vi "UE9 Synchronized Stream Example.vi"() -> ()   [LabVIEW 2021]
panel:
  out "UD Backlog B":i32
  out "UD Backlog A":i32
  in  "AIN Range":u16(ring) items=["LJ_rgBIP5V", "LJ_rgUNI5V", "LJ_rgUNI2P5V", "LJ_rgUNI1P25V", "LJ_rgUNIP625V"]
  out "Data B":dbl[][](array[numeric]) format="%.3f"
  out "Comm Backlog B":i32
  out "# Scans Read B":i32
  in  "Sync Wire Installed":bool=TRUE
  in  "Address B":string="3"
  out "Actual Scan Rate (Hz)":dbl=1000.0 format="%.3f"
  out "ms Per Loop":u32
  out "Comm Backlog A":i32
  out "# Scans Read A":i32
  out "# of iterations":i32
  out "Data A":dbl[][](array[numeric]) format="%.3f"
  in  "Scan Rate (Hz)":dbl=1000.0 format="%.3f"
  in  "Scan List":u8[](array[numeric])=[0, 1, 2, 3]
  in  "stop":bool
  in  "ConnectionType":u16(ring) items=["LJ_ctUSB", "LJ_ctETHERNET"]
  in  "Address A":string="2"
  out "Error Message":string
  in  "Resolution":i32=12
  # "Demonstrates synchronized streaming with 2 UE9s.  Connect FIO0 on unit A to FIO0 on unit B.  If the units are isolated from each other, generally\nmeaning no USB cables, you should also connect GND to GND.  Note that\tthe external clock input or output uses FIO0 in this example since no\nother timers or counters are enabled.  The external clock uses\tCounter1, so if any other timers or counters are enabled, the external\nstream clock will be on the next available FIO line, as Counter1 is always last.  If using other timer/counters, it is recommended that\nthey be configured before the stream."
  # "Specify an IP address\nfor Ethernet, or Local\nID for USB."
  # "Select if a FIO0 is connected between\nunit A and unit B.  Otherwise, the two\nunits will stream at the same time, but\nare not synchronized.  That means the\ntimes they both start streaming will\ndiffer by the time to start a stream (a\nfew milliseconds), and over time there\nwill likely be drift as the units do not\nhave the same clock."
  # "This example uses the same\nscan list for both units."
  # "(for all channels)"
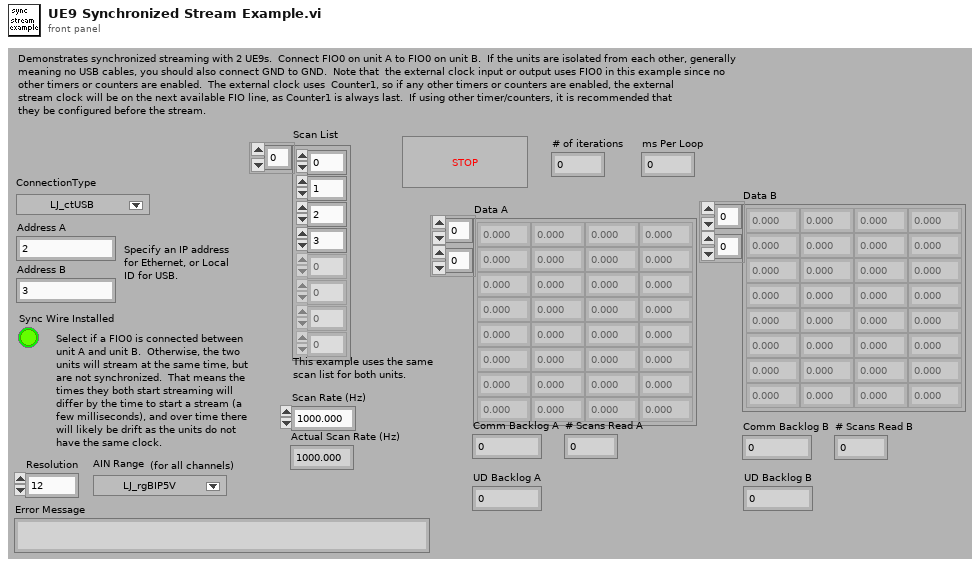
[diagram p1: front panel]
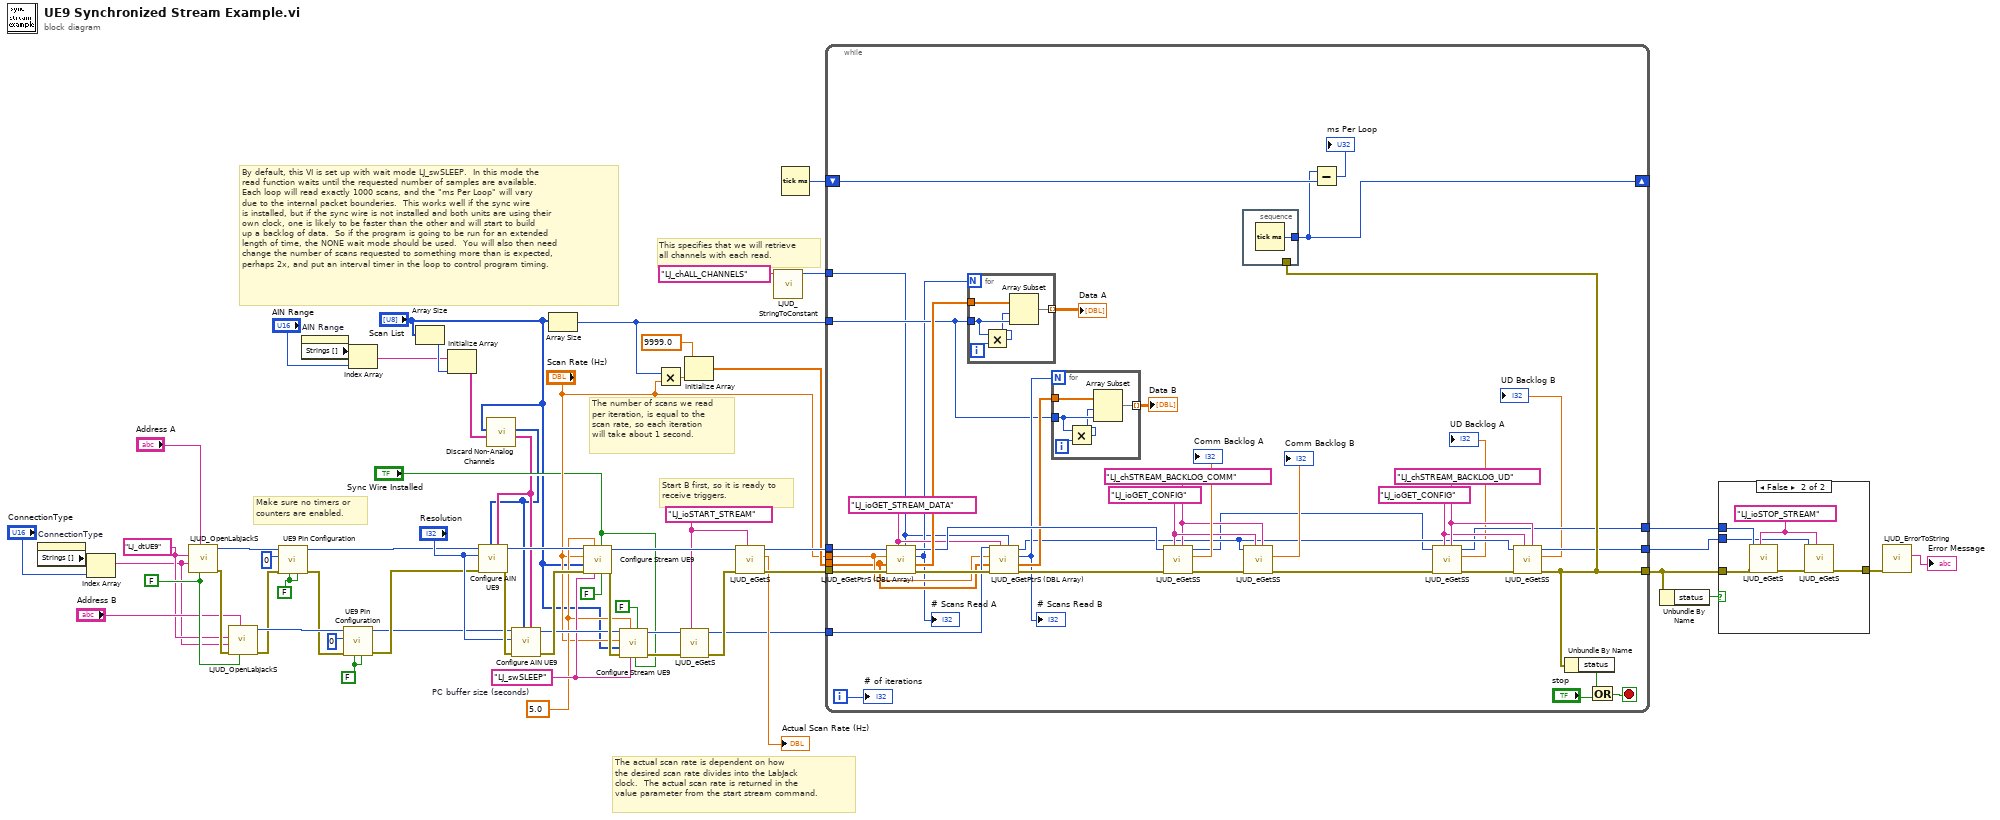
[diagram p0: block diagram]
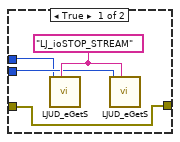
[diagram p2: hidden frame]
diagram:
  w34 = "LJ_swSLEEP" ("Wait Mode")
  w15 = "LJ_dtUE9" ("DeviceType")
  w23 = FALSE ("Enable Counter0")
  w26 = FALSE ("Enable Counter0")
  w37 = FALSE ("FirstFound")
  w33 = 5.0  # PC buffer size (seconds)
  w47 = "LJ_ioSTART_STREAM" ("IOType")
  # "This specifies that we will retrieve\nall channels with each read."
  # "Make sure no timers or\ncounters are enabled."
  # "Start B first, so it is ready to\nreceive triggers."
  # "The actual scan rate is dependent on how\nthe desired scan rate divides into the LabJack\nclock.  The actual scan rate is returned in the\nvalue parameter from the start stream command."
  # "By default, this VI is set up with wait mode LJ_swSLEEP.  In this mode the\nread function waits until the requested number of samples are available.\nEach loop will read exactly 1000 scans, and the \"ms Per Loop\" will vary\ndue to the internal packet bounderies.  This works well if the sync wire\nis installed, but if the sync wire is not installed and both units are using their\nown clock, one is likely to be faster than the other and will start to build\nup a backlog of data.  So if the program is going to be run for an extended\nlength of time, the NONE wait mode should be used.  You will also then need\nchange the number of scans requested to something more than is expected,\nperhaps 2x, and put an interval timer in the loop to control program timing."
  # "The number of scans we read\nper iteration, is equal to the\nscan rate, so each iteration\nwill take about 1 second."
  n1 = property on="ConnectionType" class="Ring (strict)"() -> ("Strings []"=w14:string[])  [unwired: 2 in, 2 out]
  n2 = Index Array(array=w14, index="ConnectionType") -> (element=w12:string)
  n3 = call "LJUD_OpenLabJackS.vi"("FirstFound"=w37, "Address"="Address A", "ConnectionType"=w12, "DeviceType"=w15) -> ("error out"=w46:errorcluster, "Handle"=w22:i32)  [unwired: 5 in, 1 out]
  n4 = call "LJUD_OpenLabJackS.vi"("FirstFound"=w37, "Address"="Address B", "error in"=w46, "ConnectionType"=w12, "DeviceType"=w15) -> ("error out"=w20:errorcluster, "Handle"=w21:i32)  [unwired: 4 in, 1 out]
  n5 = call "UE9 Pin Configuration.vi"("Enable Counter1"=w26, "Enable Counter0"=w26, "error in"=w20, "Number of Timers Enabled"=u8 0 ("# Timers Enabled"), "Handle In"=w22) -> ("error out"=w19:errorcluster, "Handle Out"=w17:i32)  [unwired: 5 in]
  n6 = property on="AIN Range" class="Ring (strict)"() -> ("Strings []"=w11:string[])  [unwired: 2 in, 2 out]
  n7 = call "UE9 Pin Configuration.vi"("Enable Counter1"=w23, "Enable Counter0"=w23, "error in"=w19, "Number of Timers Enabled"=u8 0 ("# Timers Enabled"), "Handle In"=w21) -> ("error out"=w18:errorcluster, "Handle Out"=w16:i32)  [unwired: 5 in]
  n8 = Index Array(array=w11, index="AIN Range") -> (element=w9:string)
  n9 = Array Size(array="Scan List") -> (size(s)=w48:i32)
  n10 = Initialize Array(w9, w48) -> (w4:string[])
  n11 = call "Discard Non-Analog Channels.vi"("Ranges In"=w4, "Channels In"="Scan List") -> ("Ranges Out"=w3:string[], "Channels Out"=w1:i32[])  [unwired: 6 in, 2 out]
  n12 = call "Configure AIN UE9.vi"("Ranges"=w3, "Channels"=w1, "error in"=w18, "Resolution"="Resolution", "Handle In"=w17) -> ("error out"=w45:errorcluster, "Handle Out"=w49:i32)  [unwired: 5 in]
  n13 = call "Configure AIN UE9.vi"("Ranges"=w3, "Channels"=w1, "error in"=w45, "Resolution"="Resolution", "Handle In"=w16) -> ("error out"=w44:errorcluster, "Handle Out"=w40:i32)  [unwired: 5 in]
  n14 = Array Size(array="Scan List") -> (size(s)=w54:i32)
  n15 = call "Configure Stream UE9.vi"("External Scan Trigger"=FALSE ("Scan Clock Output"), "Scan Clock Output"="Sync Wire Installed", "Wait Mode"=w34, "PC buffer size (seconds)"=w33, "error in"=w44, "Scan List"="Scan List", "Scan Rate (Hz)"="Scan Rate (Hz)", "Handle In"=w49) -> ("error out"=w42:errorcluster, "Handle Out"=w60:i32)  [unwired: 1 in, 1 out]
  n16 = call "Configure Stream UE9.vi"("External Scan Trigger"="Sync Wire Installed", "Scan Clock Output"=FALSE ("External Scan Trigger"), "Wait Mode"=w34, "PC buffer size (seconds)"=w33, "error in"=w42, "Scan List"="Scan List", "Scan Rate (Hz)"="Scan Rate (Hz)", "Handle In"=w40) -> ("error out"=w43:errorcluster, "Handle Out"=w39:i32)  [unwired: 1 in, 1 out]
  n17 = Multiply(x=w54, y="Scan Rate (Hz)") -> (x*y=w57:dbl)
  n18 = call "LJUD_eGetS.vi"("IOType"=w47, "error in"=w43, "Handle In"=w39) -> ("error out"=w41:errorcluster, "Handle Out"=w38:i32)  [unwired: 6 in, 1 out]
  n19 = Initialize Array(9999.0, w57) -> (w55:dbl[])
  n20 = call "LJUD_eGetS.vi"("IOType"=w47, "error in"=w41, "Handle In"=w60) -> ("error out"=w59:errorcluster, "Value Read"=→"Actual Scan Rate (Hz)":dbl, "Handle Out"=w58:i32)  [unwired: 6 in]
  n21 = call "LJUD_StringToConstant.vi"("String"="LJ_chALL_CHANNELS") -> ("Constant Number"=w5:i32)  [unwired: 9 in, 1 out]
  n22 = Tick Count (ms)() -> (millisecond timer value=w51:u32)
  n23 = while {
    tunnel: w5 -> [w73]
    tunnel: [w67] -> w27
    tunnel: [w64] -> w28
    tunnel: w38 -> [w82]
    shift-left: w51 -> [w94]
    shift-right: [w93] -> _
    tunnel: [w68] -> w8
    tunnel: w54 -> [w76]
    tunnel: w55 -> [w80]
    tunnel: "Scan Rate (Hz)" -> [w81]
    tunnel: w59 -> [w98]
    tunnel: w58 -> [w99]
    i -> [w95]
    stop <- w90 stop-if-true
    w71 = "LJ_ioGET_CONFIG" ("IOType")
    w72 = "LJ_chSTREAM_BACKLOG_UD" ("Channel")
    w88 = "LJ_ioGET_CONFIG" ("IOType")
    w87 = "LJ_chSTREAM_BACKLOG_COMM" ("Channel")
    w79 = "LJ_ioGET_STREAM_DATA" ("IOType")
    n24 = call "LJUD_eGetPtrS (DBL Array).vi"("Channel"=w73, "IOType"=w79, "error in"=w98, "DBL Array Write"=w80, "Value"=w81, "Handle In"=w99) -> ("error out"=w85:errorcluster, "DBL Array Read"=w97:dbl[], "Value"=w75:i32, "Handle Out"=w83:i32)  [unwired: 2 in]
    "# Scans Read A" <- w75
    n25 = for {
      N: w75 -> [_]
      tunnel: w97 -> [w112]
      tunnel: w76 -> [w111]
      tunnel: [w108] -> w96 mode=indexing
      i -> [w110]
      n26 = Multiply(x=w111, y=w110) -> (x*y=w109:i32)
      n27 = Array Subset(array=w112, index=w109, length=w111) -> (w108:dbl[])
    }
    "Data A" <- w96
    n28 = call "LJUD_eGetPtrS (DBL Array).vi"("Channel"=w73, "IOType"=w79, "error in"=w85, "DBL Array Write"=w80, "Value"=w81, "Handle In"=w82) -> ("error out"=w84:errorcluster, "DBL Array Read"=w78:dbl[], "Value"=w77:i32, "Handle Out"=w66:i32)  [unwired: 2 in]
    "# Scans Read B" <- w77
    n29 = for {
      N: w77 -> [_]
      tunnel: w78 -> [w106]
      tunnel: w76 -> [w105]
      tunnel: [w102] -> w74 mode=indexing
      i -> [w104]
      n30 = Multiply(x=w105, y=w104) -> (x*y=w103:i32)
      n31 = Array Subset(array=w106, index=w103, length=w105) -> (w102:dbl[])
    }
    "Data B" <- w74
    n32 = call "LJUD_eGetSS.vi"("Channel"=w87, "IOType"=w88, "error in"=w84, "Handle In"=w83) -> ("error out"=w89:errorcluster, "Value Read"=→"Comm Backlog A":dbl, "Handle Out"=w65:i32)  [unwired: 5 in]
    n33 = call "LJUD_eGetSS.vi"("Channel"=w87, "IOType"=w88, "error in"=w89, "Handle In"=w66) -> ("error out"=w69:errorcluster, "Value Read"=→"Comm Backlog B":dbl)  [unwired: 5 in, 1 out]
    n34 = call "LJUD_eGetSS.vi"("Channel"=w72, "IOType"=w71, "error in"=w69, "Handle In"=w65) -> ("error out"=w70:errorcluster, "Value Read"=→"UD Backlog A":dbl, "Handle Out"=w64:i32)  [unwired: 5 in]
    n35 = call "LJUD_eGetSS.vi"("Channel"=w72, "IOType"=w71, "error in"=w70, "Handle In"=w66) -> ("error out"=w68:errorcluster, "Value Read"=→"UD Backlog B":dbl, "Handle Out"=w67:i32)  [unwired: 5 in]
    n36 = stacked-sequence {
      tunnel: [w107] -> w93
      tunnel: w68 -> [_]
      frame #0 {
        n37 = Tick Count (ms)() -> (millisecond timer value=w107:u32)
      }
    }
    n38 = Subtract(x=w93, y=w94) -> (x-y=→"ms Per Loop":u32)
    n39 = Unbundle By Name(w68) -> ("status"=w100:bool)
    n40 = Or(x=w100, y="stop") -> (x .or. y?=w90:bool)
    "# of iterations" <- w95
  }
  n41 = Unbundle By Name(w8) -> ("status"=w7:bool)
  n42 = case shown="False" w7 {
    tunnel: [w113 w121] -> w52
    tunnel: w28 -> [w114 w119]
    tunnel: w27 -> [w115 w118]
    tunnel: w8 -> [w113 w117]
    frame True {
      w116 = "LJ_ioSTOP_STREAM" ("IOType")
      n43 = call "LJUD_eGetS.vi"("IOType"=w116, "Handle In"=w114) -> ()  [unwired: 7 in, 3 out]
      n44 = call "LJUD_eGetS.vi"("IOType"=w116, "Handle In"=w115) -> ()  [unwired: 7 in, 3 out]
    }
    frame False {
      w120 = "LJ_ioSTOP_STREAM" ("IOType")
      n45 = call "LJUD_eGetS.vi"("IOType"=w120, "error in"=w117, "Handle In"=w119) -> ("error out"=w122:errorcluster)  [unwired: 6 in, 2 out]
      n46 = call "LJUD_eGetS.vi"("IOType"=w120, "error in"=w122, "Handle In"=w118) -> ("error out"=w121:errorcluster)  [unwired: 6 in, 2 out]
    }
  }
  n47 = call "LJUD_ErrorToString.vi"("error in"=w52) -> ("String"=→"Error Message":string)  [unwired: 10 in]
